vi "Read Ghosts Pictures.vi"(8 "error in (no error)":errorcluster, 11 "Ghosts in":refnum<class "Ghosts.lvclass">) -> (0 "error out":errorcluster, 2 "Ghosts Pictures":T1, 3 "Ghosts out":refnum<class "Ghosts.lvclass">)   [LabVIEW 2016]
uses:
  Ghosts.lvclass
  C:/Users/lucamach/Documents/SE/Learning OOP/PacMan/PacMan Classes/Geometric Figure/UI Object.lvclass
  Generic Controls/Ghost Pictures.ctl
  PacManClasses.lvlib
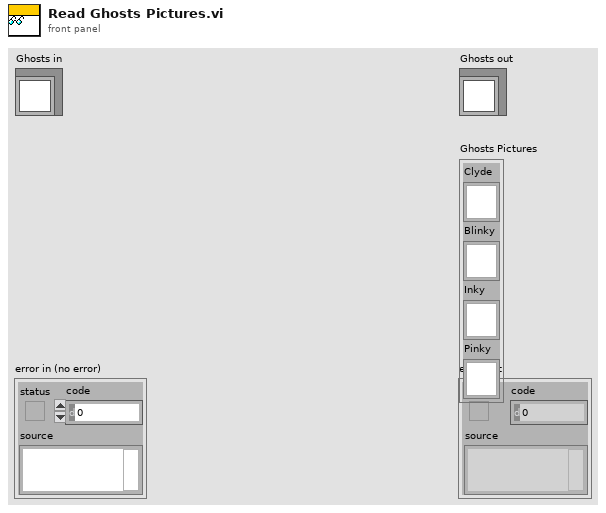
[diagram p1: front panel]
types:
  T1 = typedef "PacManClasses.lvlib/Ghost Pictures.ctl" = cluster{"Clyde":picture, "Blinky":picture, "Inky":picture, "Pinky":picture}
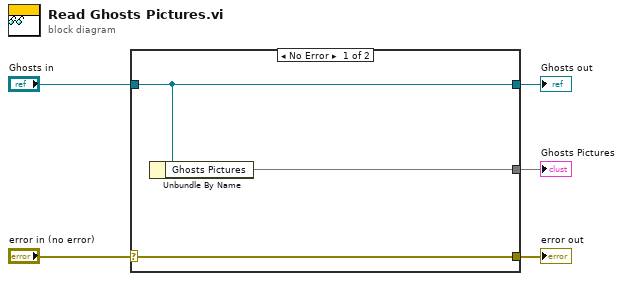
[diagram p0: block diagram]
diagram:
  n1 = case shown="No Error" "error in (no error)" {
    selector: "error in (no error)" -> [w8 w9]
    tunnel: [w8 w9] -> w4
    tunnel: [w7 w10] -> w2
    tunnel: "Ghosts in" -> [w7 w10]
    tunnel: [w6 _] -> w1
    frame No Error {
      n2 = Unbundle By Name(w7) -> ("Ghosts Pictures"=w6)
    }
    frame Error {
    }
  }
  "error out" <- w4
  "Ghosts out" <- w2
  "Ghosts Pictures" <- w1
